vi "MPM_Set_Mode.vi"(8 "error in (no error)":errorcluster, 10 "mode":i32(ring) items=["ManualRangeConstant", "ManualRangeSweep", "AutoRangeConstant", "AutoRangeSweep", "Freerun"], 11 ".NET Reference in":refnum<k24>) -> (0 "error out":errorcluster, 3 "Reference out":refnum<k24>)   [LabVIEW 2017]
uses:
  C:/Users/Ssantec_Test/Documents/Instrument_DLL_Sample_Labview_20220902_Ver1.2.2/DLL/x86/InstrumentDLL.dll
  DLL/x86/InstrumentDLL.dll
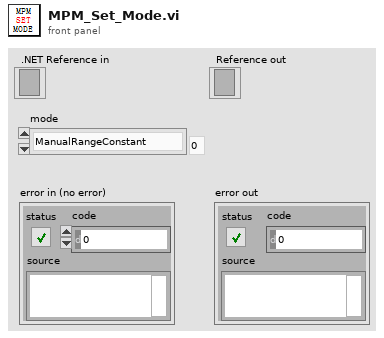
[diagram p1: front panel]
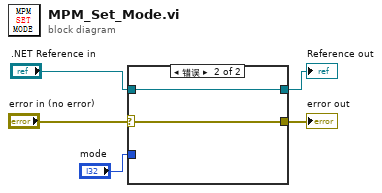
[diagram p0: block diagram]
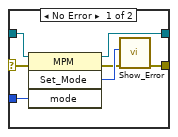
[diagram p2: hidden frame]
diagram:
  n1 = case shown="错误" "error in (no error)" {
    selector: "error in (no error)" -> [w6 w13]
    tunnel: ".NET Reference in" -> [w12 w14]
    tunnel: [w11 w14] -> w4
    tunnel: "mode" -> [w10 _]
    tunnel: [w7 w13] -> w2
    frame No Error {
      n2 = invoke class="MPM" method="Set_Mode"(reference=w12, error in=w6, "mode"=w10) -> (reference out=w11:refnum<k24>, error out=w8:errorcluster, "Set_Mode"=w9:i32)  [unwired: 1 in, 1 out]
      n3 = call "Show_Error.vi"("error in (no error)"=w8, "Error"=w9) -> ("error out"=w7:errorcluster)  [unwired: 9 in]
    }
    frame Error {
    }
  }
  "Reference out" <- w4
  "error out" <- w2
